vi "SPI Full Engine.vi"(8 "error in (no error)":errorcluster, 11 "All SPI Settings":T1={"SPI Signal Settings"={"SCLK"={"Signal"="sbRIO-9651 Socket\\PMOD1_Pin4_out", "Signal_Enable"="sbRIO-9651 Socket\\PMOD1_Pin4_enable", "Output?"=FALSE}, "Signal Settings"={"MISO"="sbRIO-9651 Socket\\PMOD1_Pin3_in", "Signal_Enable"="sbRIO-9651 Socket\\PMOD1_Pin4_enable", "Output?"=FALSE}, "MOSI"={"Signal"="sbRIO-9651 Socket\\PMOD1_Pin4_out", "Signal_Enable"="sbRIO-9651 Socket\\PMOD1_Pin4_enable", "Output?"=FALSE}, "CS0"={"Signal"="sbRIO-9651 Socket\\PMOD1_Pin4_out", "Signal_Enable"="sbRIO-9651 Socket\\PMOD1_Pin4_enable", "Output?"=FALSE}, "CS1"={"Signal"="sbRIO-9651 Socket\\PMOD1_Pin4_out", "Signal_Enable"="sbRIO-9651 Socket\\PMOD1_Pin4_enable", "Output?"=FALSE}, "CS2"={"Signal"="sbRIO-9651 Socket\\PMOD1_Pin4_out", "Signal_Enable"="sbRIO-9651 Socket\\PMOD1_Pin4_enable", "Output?"=FALSE}, "CS3"={"Signal"="sbRIO-9651 Socket\\PMOD1_Pin4_out", "Signal_Enable"="sbRIO-9651 Socket\\PMOD1_Pin4_enable", "Output?"=FALSE}, "CS4"={"Signal"="sbRIO-9651 Socket\\PMOD1_Pin4_out", "Signal_Enable"="sbRIO-9651 Socket\\PMOD1_Pin4_enable", "Output?"=FALSE}, "CS5"={"Signal"="sbRIO-9651 Socket\\PMOD1_Pin4_out", "Signal_Enable"="sbRIO-9651 Socket\\PMOD1_Pin4_enable", "Output?"=FALSE}}, "SPI Internal Signals"={"DLU To SPI Engine Data FIFO"="DLU To SPI Engine Data", "SPI Engine to DLU Data FIFO"="SPI Engine to DLU Data", "Data to SPI Engine (Cache) Register"="Data to SPI Engine (Cache)", "SPI PHY Settings to SPI Engine (Cahche) Register"="SPI PHY Settings to SPI Engine (Cache)"}, "SPI PHY Settings"={"Divide Value"=0, "Transfer Length (bits)"=0, "CS Asserted Polarity"=FALSE, "Clock Polarity (CPOL)"=FALSE, "Clock Phase (CPHA)"=FALSE, "Lengthen MISO Setup"=FALSE, "Direction Change Bit"=0, "MOSI Starts as Output"=FALSE, "Tristatable MOSI"=FALSE}, "SPI Engine Source"="120MHz"} {"SPI PHY Settings"."Direction Change Bit" max=64 step=1; "SPI PHY Settings"."Transfer Length (bits)" min=1 max=64 step=1}) -> ()   [LabVIEW 2014]
uses:
  Controls/All SPI Settings.ctl
  Controls/SPI Settings.ctl
  Controls/Signal Properties.ctl
  Controls/Internal Data (SPI API).ctl
  <userlib>/_NI SPI IP/FPGA/Controllers/Public/Transfer Settings.ctl
  <vilib>/Platform/TimedLoop/XDataNode/timing_clust.ctl
  <vilib>/Platform/TimedLoop/XDataNode/nitl_modes.ctl
  <vilib>/Platform/TimedLoop/XDataNode/wakeup.ctl
  <vilib>/rvi/Emulation/niFpgaSctlEmulationGetInTimedLoop.vi
  <vilib>/rvi/Emulation/niFpgaEmulationReportErrorSimple.vi
  <vilib>/rvi/Emulation/niFpgaGetClockAttributes.vi
  <vilib>/rvi/Emulation/niFpgaCriticalErrorInLSC.vi
  <vilib>/Platform/TimedLoop/XDataNode/XDataNode.xnode
  <vilib>/Platform/TimedLoop/XDataNode/XDNodeRunTimeDep.lvlib
  <userlib>/_NI SPI IP/FPGA/Controllers/NI SPI IP FPGA.lvlib
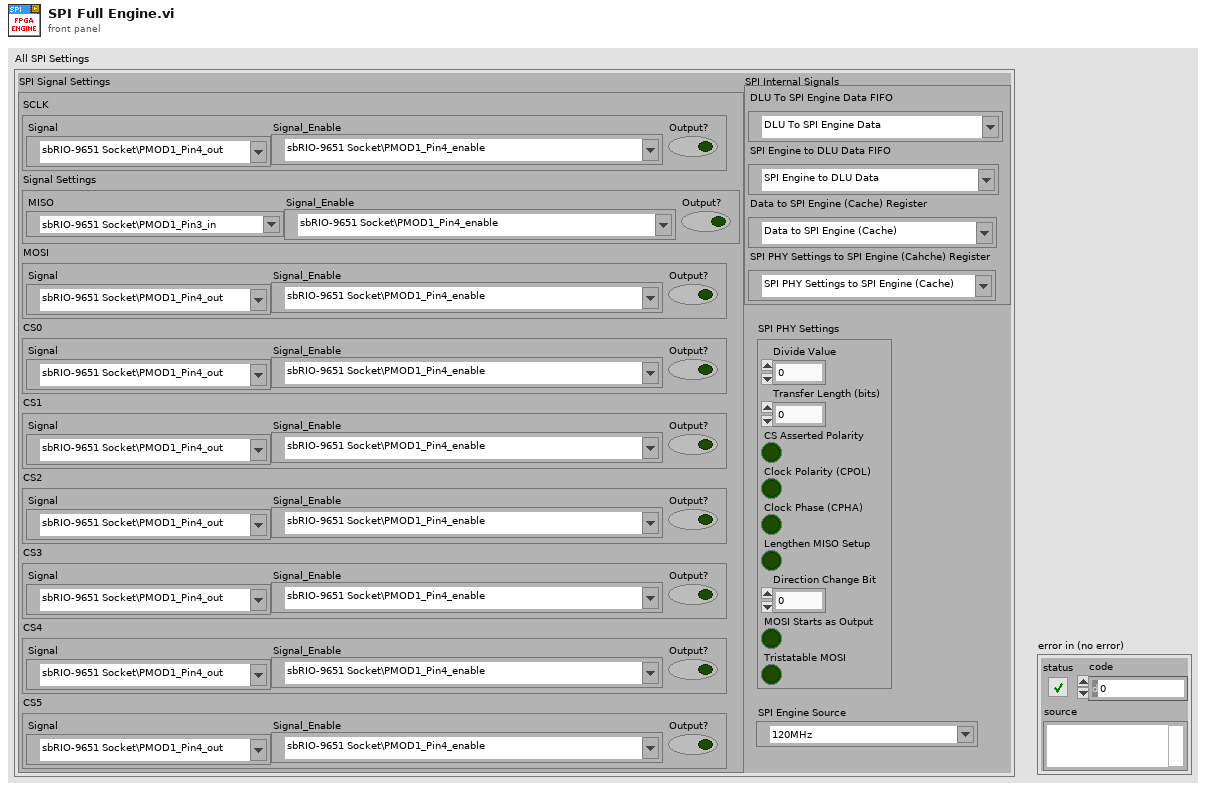
[diagram p1: front panel]
types:
  T1 = typedef "All SPI Settings.ctl" = cluster{"SPI Signal Settings":T2, "SPI Internal Signals":T4, "SPI PHY Settings":T5, "SPI Engine Source":refnum<k21>}
  T2 = typedef "SPI Settings.ctl" = cluster{"SCLK":T3, "Signal Settings":cluster{"MISO":refnum<k21>, "Signal_Enable":refnum<k21>, "Output?":bool}, "MOSI":T3, "CS0":T3, "CS1":T3, "CS2":T3, "CS3":T3, "CS4":T3, "CS5":T3}
  T3 = typedef "Signal Properties.ctl" = cluster{"Signal":refnum<k21>, "Signal_Enable":refnum<k21>, "Output?":bool}
  T4 = typedef "Internal Data (SPI API).ctl" = cluster{"DLU To SPI Engine Data FIFO":refnum<k21>, "SPI Engine to DLU Data FIFO":refnum<k21>, "Data to SPI Engine (Cache) Register":refnum<k21>, "SPI PHY Settings to SPI Engine (Cahche) Register":refnum<k21>}
  T5 = typedef "NI SPI IP FPGA.lvlib/Transfer Settings.ctl" = cluster{"Divide Value":u8, "Transfer Length (bits)":u8, "CS Asserted Polarity":bool, "Clock Polarity (CPOL)":bool, "Clock Phase (CPHA)":bool, "Lengthen MISO Setup":bool, "Direction Change Bit":u8, "MOSI Starts as Output":bool, "Tristatable MOSI":bool}
  T6 = typedef "SPI DIO Enable Lines.ctl" = cluster{"SCLK_en":refnum<k21>, "MISO_en":refnum<k21>, "MOSI_en":refnum<k21>, "CS0_en":refnum<k21>, "CS1_en":refnum<k21>, "CS2_en":refnum<k21>, "CS3_en":refnum<k21>, "CS4_en":refnum<k21>, "CS5_en":refnum<k21>}
  T7 = typedef "SPI Digital IO Lines.ctl" = cluster{"SCLK":refnum<k21>, "MISO":refnum<k21>, "MOSI":refnum<k21>, "CS 0":refnum<k21>, "CS 1":refnum<k21>, "CS 2":refnum<k21>, "CS 3":refnum<k21>, "CS 4":refnum<k21>, "CS 5":refnum<k21>}
  T8 = typedef "XDNodeRunTimeDep.lvlib/timing_clust.ctl" = cluster{"Expected End [f-1]":u64, "Actual End [f-1]":u64, "Finished Late? [f-1]":bool, "Expected End [i-1]":u64, "Actual End [i-1]":u64, "Finished Late? [i-1]":bool, "Expected Start [i]":u64, "Actual Start [i]":u64, "Expected Start [f]":u64, "Actual Start [f]":u64, "Source Name":string, "Structure Name":string, "Period":i64, "Deadline":i64, "Offset":i64, "Start":i64, "Priority":i32, "Timeout":i32, "Mode":T9, "Wakeup Reason":T10, "Error":errorcluster, "Source Type":string, "Secondary Source Type":string, "Global End Time":u64, "Global Start Time":u64, "Frame Duration":u64, "Iteration Duration":u64, "Assigned CPU":i32, "I/O Scan Engine Mode":u32}
  T9 = typedef "XDNodeRunTimeDep.lvlib/nitl_modes.ctl" = enum32{"No Change", "Process missed periods, maintain original phase", "Discard missed periods, maintain original phase", "Process missed periods, ignore original phase", "Discard missed periods, ignore original phase"}
  T10 = typedef "XDNodeRunTimeDep.lvlib/wakeup.ctl" = enum32{"Normal", "Aborted", "Asynchronous wakeup", "Timing source error", "Timed loop error", "Timeout"}
  T11 = typedef "NI SPI IP FPGA.lvlib/Spi Master Inputs.ctl" = cluster{"MISO":bool}
  T12 = typedef "NI SPI IP FPGA.lvlib/Spi Master Outputs.ctl" = cluster{"Chip Select":bool, "Clock":bool, "MOSI":bool, "MOSI OE":bool}
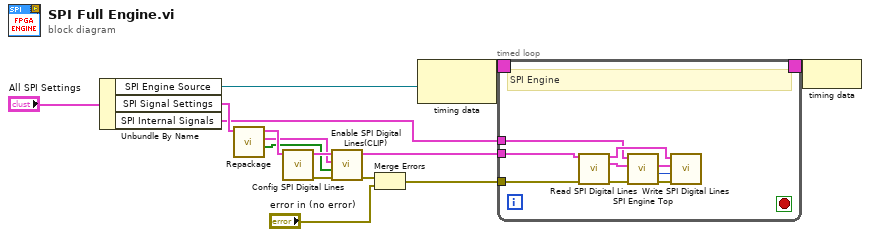
[diagram p0: block diagram]
diagram:
  n1 = Unbundle By Name("All SPI Settings") -> ("SPI Engine Source"=w1:refnum<k21>, "SPI Signal Settings"=w3:T2, "SPI Internal Signals"=w2:T4)
  n2 = call "Repackage.vi"("SPI Settings"=w3) -> ("Enable"=w6:bool[], "Enable Lines"=w5:T6, "Chip Select DIO Lines"=w7:T7)  [unwired: 8 in]
  n3 = call "Config SPI Digital Lines.vi"("SPI DIO Lines"=w7) -> ("error out"=w13:errorcluster, "Chip Select DIO Lines"=w12:T7)  [unwired: 9 in]
  n4 = call "Enable SPI Digital Lines(CLIP).vi"("error in"=w13, "Enable"=w6, "Enable Lines"=w5, "SPI DIO Lines"=w12) -> ("error out"=w11:errorcluster, "Chip Select DIO Lines"=w10:T7)  [unwired: 6 in]
  n5 = Merge Errors(w11, "error in (no error)") -> (w9:errorcluster)
  n6 = node-c288(w1) -> (w15:T8)
  n7 = timed-loop {
    tunnel: w2 -> [w21]
    tunnel: w9 -> [w19]
    tunnel: w10 -> [w23]
    timing: w15 -> [_]
    timing-out: [_] -> w14
    stop <- _ stop-if-true
    # "SPI Engine"
    n8 = call "Read SPI Digital Lines.vi"("Chip Select DIO Lines"=w23, "error in"=w19) -> ("Chip Select DIO Lines Out"=w24:T7, "SPI Read Data"=w20:T11, "error out"=w18:errorcluster)  [unwired: 11 in]
    n9 = call "SPI Engine Top.vi"("error in"=w18, "SPI Read Data"=w20, "SPI API References"=w21) -> ("error out"=w17:errorcluster, "Chip Select ID"=w16:u8, "SPI DIO Output"=w22:T12)  [unwired: 5 in, 1 out]
    n10 = call "Write SPI Digital Lines.vi"("error in"=w17, "CS Index"=w16, "spi output"=w22, "Chip Select DIO Lines"=w24) -> ()  [unwired: 6 in, 2 out]
  }
  n11 = node-c288(w14) -> ()
